vi "Init Hardware.vi"(8 "error in (no error)":errorcluster, 11 "LakeShore 370 Driver in":refnum<class "LakeShore 370 Driver.lvclass">) -> (0 "error out":errorcluster, 3 "LakeShore 370 Driver out":refnum<class "LakeShore 370 Driver.lvclass">)   [LabVIEW 2016, in "LakeShore 370 Driver.lvclass"]
uses:
  LakeShore 370 Driver.lvclass
  C:/github/NHMFL_Core/Libraries/Instruments/Instrument Driver/Instrument Driver.lvclass
  Instrument Driver/Instrument Driver.lvclass/Instrument Driver.ctl
  Instrument Driver/Read Recorder name.vi
  Instrument Driver/Write Channel names.vi
  Instrument Driver/Write Channel units.vi
  Simple VISA Reader/Simple VISA Reader Driver.lvclass
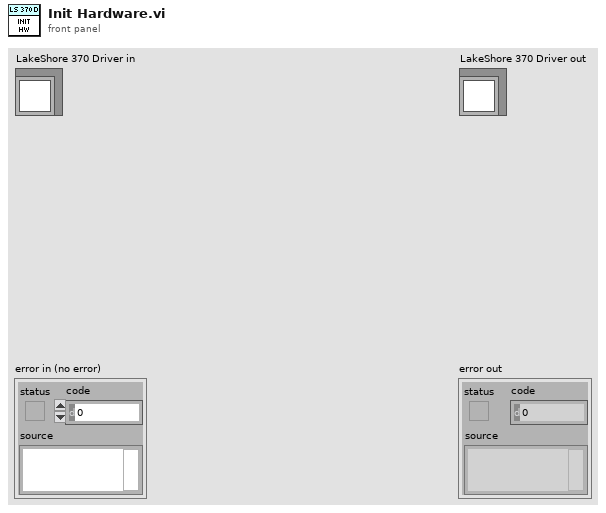
[diagram p1: front panel]
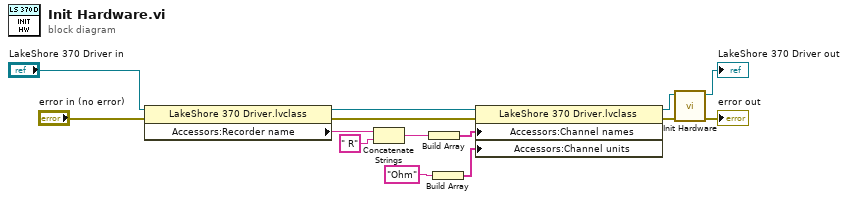
[diagram p0: block diagram]
diagram:
  n1 = property class="LakeShore 370 Driver.lvclass"(reference="LakeShore 370 Driver in", error in="error in (no error)") -> (reference out=w5:refnum<class "LakeShore 370 Driver.lvclass">, error out=w3:errorcluster, "Accessors:Recorder name"=w1:string)
  n2 = Concatenate Strings(w1, " R") -> (w2:string)
  n3 = Build Array(w2) -> (w10:string[])
  n4 = Build Array("Ohm") -> (w8:string[])
  n5 = property class="LakeShore 370 Driver.lvclass"(reference=w5, error in=w3, "Accessors:Channel names"=w10, "Accessors:Channel units"=w8) -> (reference out=w12:refnum<class "LakeShore 370 Driver.lvclass">, error out=w7:errorcluster)
  n6 = call-parent "Init Hardware.vi"("error in (no error)"=w7, "Instrument Driver in"=w12) -> ("error out"=→"error out":errorcluster, "Instrument Driver out"=→"LakeShore 370 Driver out":refnum<class "LakeShore 370 Driver.lvclass">)  [unwired: 8 in]
